vi "Wf_to_STFT.vi"(6 "STFT Config":T2={"FFT block size"=1024, "window"=1, "time segment"={"from [s]"=-1.0, "to [s]"=-1.0, "time increment"=20.0, "time increment units (%)"=enum."%"}, "dB On (T)"=TRUE, "Dynamic Range(dB)"=80.0, "Mel?"=TRUE} {"window" items=["None "=0, "Hanning"=1, "Hamming"=2, "Blackman-Harris"=3, "Exact Blackman"=4, "Blackman"=5, "Flat Top"=6, "4 Term B-Harris "=7, "7 Term B-Harris"=8, "Low Sidelobe"=9, "Blackman Nuttall"=11]}, 8 "error in (no error)":errorcluster, 11 "WF":waveform(dbl)) -> (0 "error out":errorcluster, 1 "STFT":T1, 3 "Image_data":u8[][](array[numeric]))   [LabVIEW 2020]
uses:
  Controls/Wave2STFT_Cfg.ctl
  <vilib>/Analysis/2dsp.llb/Power Spectrum (DBL).vi
  Freq2Mel.vi
  Meel2Freq(1D).vi
  <vilib>/Analysis/NI_AALPro.lvlib
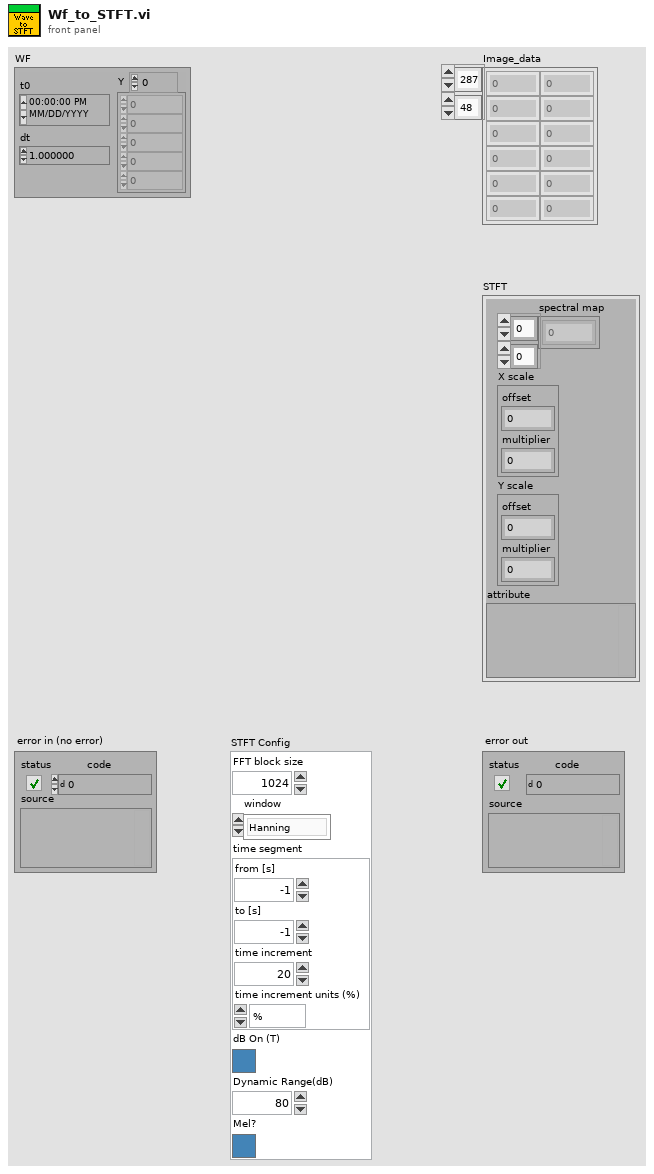
[diagram p1: front panel]
types:
  T1 = cluster{"spectral map":dbl[][], "X scale":cluster{"offset":dbl, "multiplier":dbl}, "Y scale":cluster{"offset":dbl, "multiplier":dbl}, "attribute":variant}
  T2 = typedef "Wave2STFT_Cfg.ctl" = cluster{"FFT block size":i32, "window":u16, "time segment":cluster{"from [s]":dbl, "to [s]":dbl, "time increment":dbl, "time increment units (%)":enum16{"%", "s", "ms"}}, "dB On (T)":bool, "Dynamic Range(dB)":sgl, "Mel?":bool}
  T3 = cluster{"from [s]":dbl, "to [s]":dbl, "time increment":dbl, "time increment units (%)":enum16{"%", "s", "ms"}}
  T4 = cluster{"FFT block size":i32, "number of FFT":i32, "start index":i32, "increment":dbl}
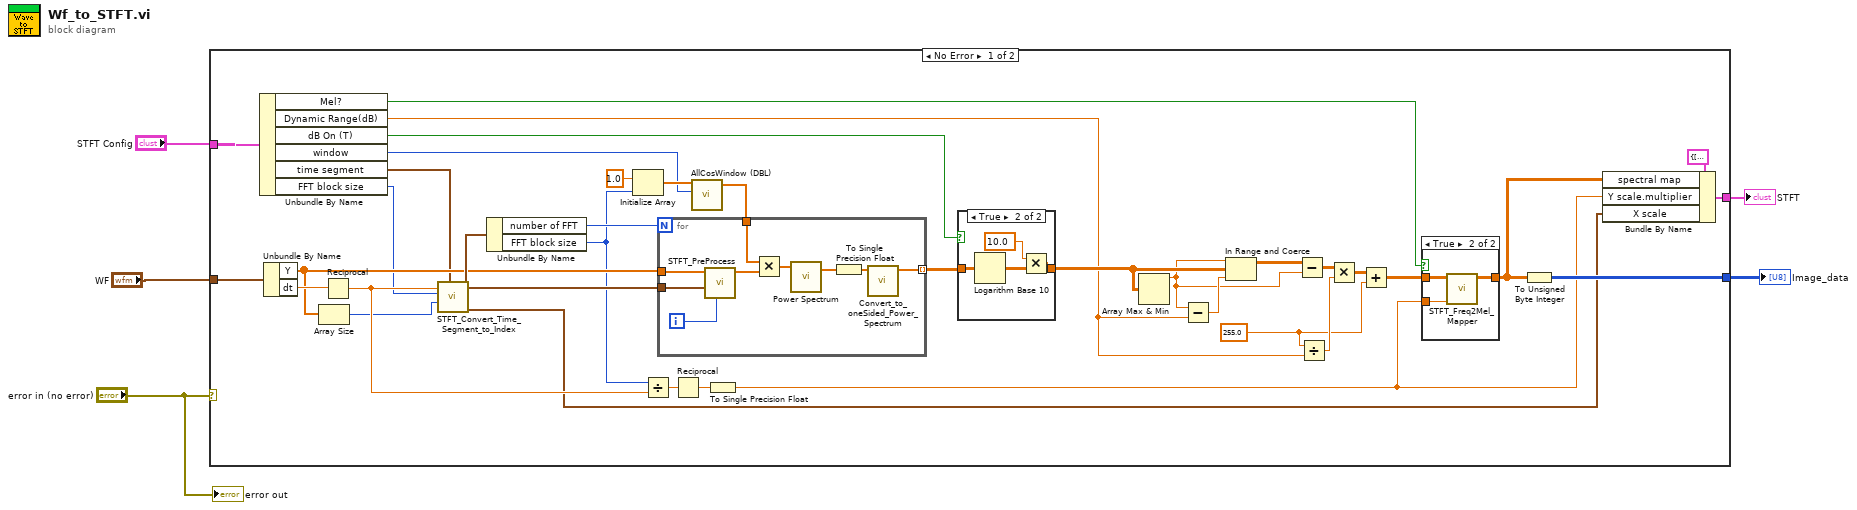
[diagram p0: block diagram]
diagram:
  n1 = case shown="No Error" "error in (no error)" {
    tunnel: "STFT Config" -> [w41 _]
    tunnel: [w11 _] -> w4
    tunnel: [w10 _] -> w3
    tunnel: "WF" -> [w6 _]
    frame No Error {
      w35 = sgl 255.0 ("x")
      n2 = Unbundle By Name(w41) -> ("Mel?"=w23:bool, "Dynamic Range(dB)"=w21:sgl, "dB On (T)"=w13:bool, "window"=w16:u16, "time segment"=w14:T3, "FFT block size"=w15:i32)
      n3 = Unbundle By Name(w6) -> ("Y"=w25:dbl[], "dt"=w30:dbl)
      n4 = Array Size(array=w25) -> (size(s)=w24:i32)
      n5 = Reciprocal(x=w30) -> (1/x=w27:dbl)
      n6 = call "STFT_Convert_Time_Segment_to_Index.vi"("time segment"=w14, "Samples"=w24, "FFT block size"=w15, "sampling frequency [Hz]"=w27) -> ("to and delta t [s]"=w8:cluster{"to":dbl, "delta t":dbl}, "FFT info"=w29:T4)  [unwired: 6 in]
      n7 = Unbundle By Name(w29) -> ("number of FFT"=w28:i32, "FFT block size"=w19:i32)
      n8 = Initialize Array(1.0 ("element"), w19) -> (w18:dbl[])
      n9 = Divide(x=w19, y=w27) -> (x/y=w32:dbl)
      n10 = Reciprocal(x=w32) -> (1/x=w31:dbl)
      n11 = call <vilib>:"AllCosWindow (DBL).vi"("window"=w16, "X"=w18) -> ("Windowed X"=w17:dbl[])  [unwired: 3 in, 1 out]
      n12 = for {
        N: w28 -> [_]
        tunnel: w25 -> [w50]
        tunnel: w29 -> [w46]
        tunnel: [w48] -> w26 mode=indexing
        tunnel: w17 -> [w43]
        i -> [w49]
        n13 = call "STFT_PreProcess.vi"("iteration"=w49, "FFT info"=w46, "Signal in"=w50) -> ("preprocessed Signal out"=w42:dbl[])  [unwired: 8 in]
        n14 = Multiply(x=w43, y=w42) -> (x*y=w44:dbl[])
        n15 = call-poly <vilib>:"Power Spectrum.vi"("X"=w44) -> ("Power Spectrum"=w47:dbl[])  [unwired: 1 out]
        n16 = To Single Precision Float(number=w47) -> (single precision float=w45:sgl[])
        n17 = call "Convert_to_oneSided_Power_Spectrum.vi"("two-sided power spectrum"=w45) -> ("one-sided power spectrum"=w48:sgl[])  [unwired: 9 in, 1 out]
      }
      n18 = To Single Precision Float(number=w31) -> (single precision float=w9:sgl)
      n19 = case shown="True" w13 {
        tunnel: w26 -> [w51 w55]
        tunnel: [w51 w52] -> w34
        frame False {
        }
        frame True {
          n20 = Logarithm Base 10(1:w55) -> (0:w53:sgl[][])
          n21 = Multiply(x=sgl 10.0 ("y"), y=w53) -> (x*y=w52:sgl[][])
        }
      }
      n22 = Array Max & Min(array=w34) -> (max value=w22:sgl)  [unwired: 3 out]
      n23 = Subtract(x=w22, y=w21) -> (x-y=w36:sgl)
      n24 = In Range and Coerce(upper limit=w22, x=w34, lower limit=w36) -> (coerced(x)=w37:sgl[][])  [unwired: 1 out]
      n25 = Subtract(x=w37, y=w22) -> (x-y=w39:sgl[][])
      n26 = Divide(x=w35, y=w21) -> (x/y=w38:sgl)
      n27 = Multiply(x=w39, y=w38) -> (x*y=w40:sgl[][])
      n28 = Add(x=w40, y=w35) -> (x+y=w33:sgl[][])
      n29 = case shown="True" w23 {
        tunnel: w33 -> [w56 w59]
        tunnel: [w56 w58] -> w7
        tunnel: w9 -> [_ w57]
        frame False {
        }
        frame True {
          n30 = call "STFT_Freq2Mel_Mapper.vi"("df"=w57, "spectral map"=w59) -> ("spectral map out"=w58:sgl[][])  [unwired: 9 in]
        }
      }
      n31 = To Unsigned Byte Integer(number=w7) -> (unsigned 8bit integer=w10:u8[][])
      n32 = Bundle By Name(cluster=T1 {"spectral map"=[], "X scale"={"offset"=0.0, "multiplier"=0.0}, "Y scale"={"offset"=0.0, "multiplier"=0.0}, "attribute"=variant} ("STFT"), "spectral map"=w7, "Y scale.multiplier"=w9, "X scale"=w8) -> (w11:T1)
    }
    frame Error {
    }
  }
  "Image_data" <- w3
  "STFT" <- w4
  "error out" <- "error in (no error)"
